vi "ManualTresholdControlL0.vi"() -> ()   [LabVIEW 2012]
panel:
  in  "Treshold":i16(slide) min=0 max=1000 scale=0.0..1000.0
  in  "stop":bool
  in  "Channel":i8
  out "error out":errorcluster
  in  "error in":errorcluster
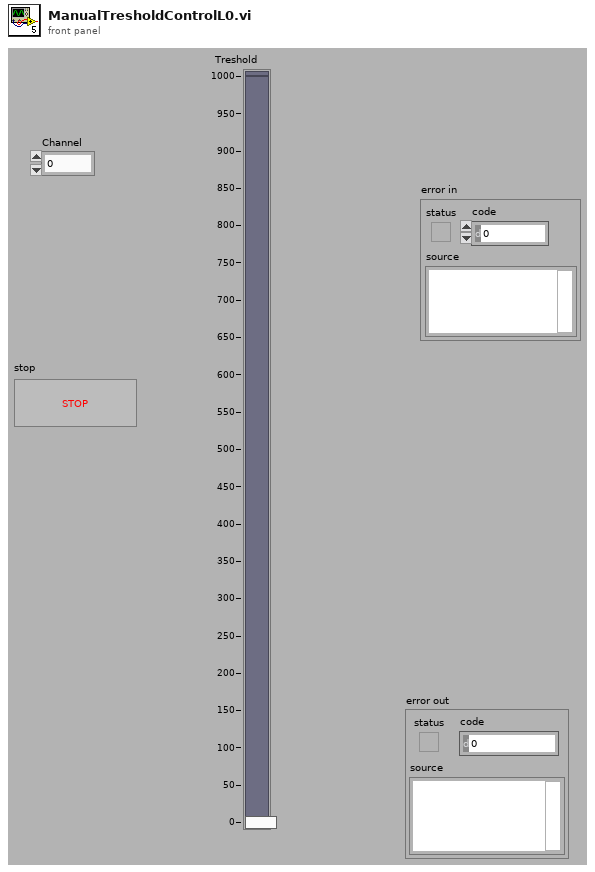
[diagram p1: front panel]
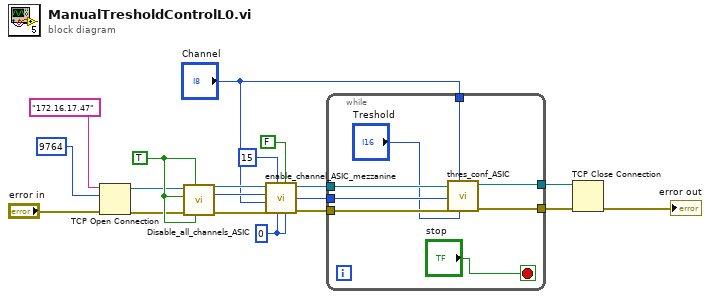
[diagram p0: block diagram]
diagram:
  w13 = u32 0 ("Ib_clipVb")
  w14 = TRUE ("Att_en_b")
  n1 = TCP Open Connection(address="172.16.17.47", remote port or service name=u16 9764, error in (no error)="error in") -> (connection ID=w4:refnum<k5>, error out=w5:errorcluster)  [unwired: 2 in]
  n2 = call "Disable_all_channels_ASIC.vi"("CompBuf_en_b"=w14, "Att_en_b"=w14, "error in"=w5, "Clip_en_b"=w14, "connection ID"=w4) -> ("error out"=w16:errorcluster, "id_out"=w11:i32, "connection ID out"=w15:refnum<k5>)  [unwired: 4 in]
  n3 = call "enable_channel_ASIC_mezzanine.vi"("Clip_sel_b"=w13, "maj/sum"=FALSE, "Ib_clipVb"=w13, "Att gain"=u32 15, "error in"=w16, "Channel"="Channel", "id_in"=w11, "connection ID"=w15) -> ("error out"=w9:errorcluster, "id_out"=w3:i32, "connection ID out"=w8:refnum<k5>)  [unwired: 1 in]
  n4 = while {
    tunnel: w9 -> [w27]
    tunnel: w8 -> [w26]
    tunnel: [w25] -> w7
    tunnel: [w24] -> w6
    tunnel: w3 -> [w23]
    tunnel: "Channel" -> [w22]
    stop <- "stop" stop-if-true
    n5 = call "thres_conf_ASIC.vi"("threshold"="Treshold", "Ring"=w22, "error out 3"=w27, "Id in"=w23, "connection ID"=w26) -> ("error out 2"=w25:errorcluster, "connection ID out"=w24:refnum<k5>)  [unwired: 3 in, 2 out]
  }
  n6 = TCP Close Connection(connection ID=w6, error in (no error)=w7) -> (error out=→"error out":errorcluster)  [unwired: 1 in, 1 out]
